vi "Display.vi"(0 "reference in":refnum<class "ForecastConditionDisplay.lvclass">, 5 "error in (no error)":errorcluster) -> (14 "reference out":refnum<class "ForecastConditionDisplay.lvclass">, 16 "WeatherData":T1, 19 "error out":errorcluster)   [LabVIEW 2010, in "ForecastConditionDisplay.lvclass"]
uses:
  ForecastConditionDisplay.lvclass
  WeatherData.ctl
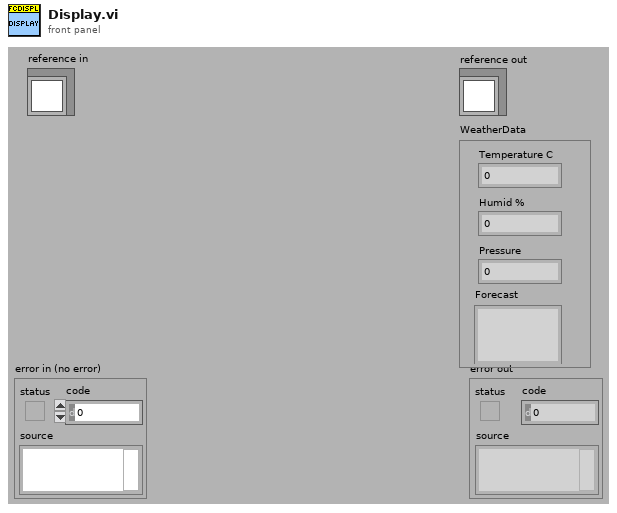
[diagram p1: front panel]
types:
  T1 = typedef "WeatherData.ctl" = cluster{"Temperature C":dbl, "Humid %":dbl, "Pressure":dbl, "Forecast":string}
  T2 = typedef "ForecastConditionDisplay.lvclass/ObjectAttributes.ctl" = cluster{"WeatherData":T1}
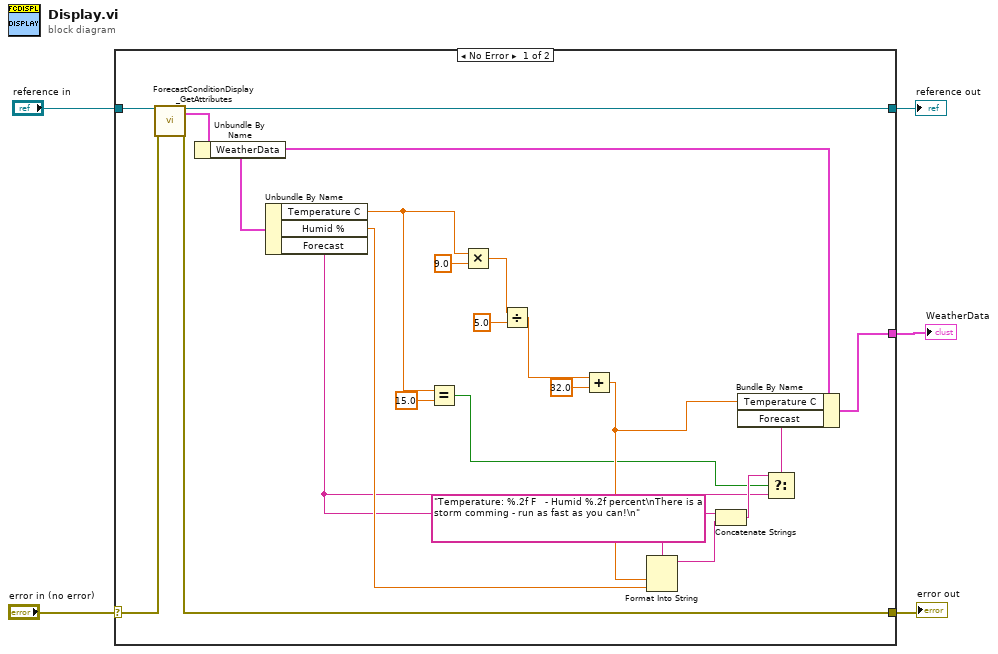
[diagram p0: block diagram]
diagram:
  n1 = case shown="No Error" "error in (no error)" {
    selector: "error in (no error)" -> [w27 w29]
    tunnel: [w25 w29] -> w4
    tunnel: [w23 w28] -> w2
    tunnel: "reference in" -> [w24 w28]
    tunnel: [w16 _] -> w1
    frame No Error {
      n2 = call "ForecastConditionDisplay_GetAttributes.vi"("reference in"=w24, "error in (no error)"=w27) -> ("reference out"=w23:refnum<class "ForecastConditionDisplay.lvclass">, "Data"=w26:T2, "error out"=w25:errorcluster)  [unwired: 14 in, 1 out]
      n3 = Unbundle By Name(w26) -> ("WeatherData"=w17:T1)
      n4 = Unbundle By Name(w17) -> ("Temperature C"=w11:dbl, "Humid %"=w13:dbl, "Forecast"=w7:string)
      n5 = Equal?(x=w11, y=15.0) -> (x = y?=w8:bool)
      n6 = Multiply(x=w11, y=9.0) -> (x*y=w21:dbl)
      n7 = Divide(x=w21, y=5.0) -> (x/y=w19:dbl)
      n8 = Add(x=w19, y=32.0) -> (x+y=w14:dbl)
      n9 = Format Into String(format string="Temperature: %.2f F   - Humid %.2f percent\nThere is a storm comming - run as fast as you can!\n", w14, w13) -> (resulting string=w12:string)  [unwired: 2 in, 1 out]
      n10 = Concatenate Strings(w7, w12) -> (w9:string)
      n11 = Select(t=w9, s=w8, f=w7) -> (s? t:f=w6:string)
      n12 = Bundle By Name(cluster=w17, "Temperature C"=w14, "Forecast"=w6) -> (w16:T1)
    }
    frame Error {
    }
  }
  "error out" <- w4
  "reference out" <- w2
  "WeatherData" <- w1
